vi "Write.vi"(7 "Input String":string, 8 "error in (no error)":errorcluster, 11 "VISA resource name":refnum<visa-resource-name>) -> (0 "error out":errorcluster, 2 "String":string, 3 "VISA resource name out":refnum<visa-resource-name>)   [LabVIEW 2021, in "BK Precision 169XB.lvlib"]
uses:
  BK Precision 169XB.lvlib
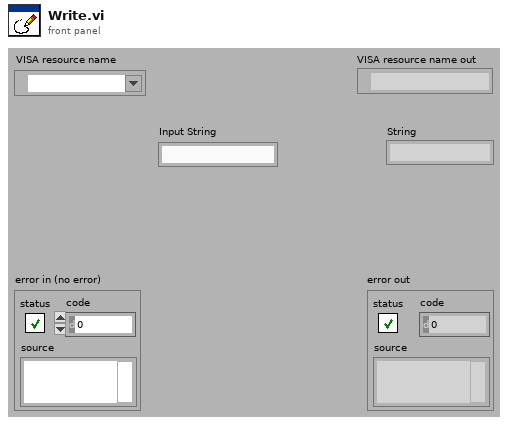
[diagram p1: front panel]
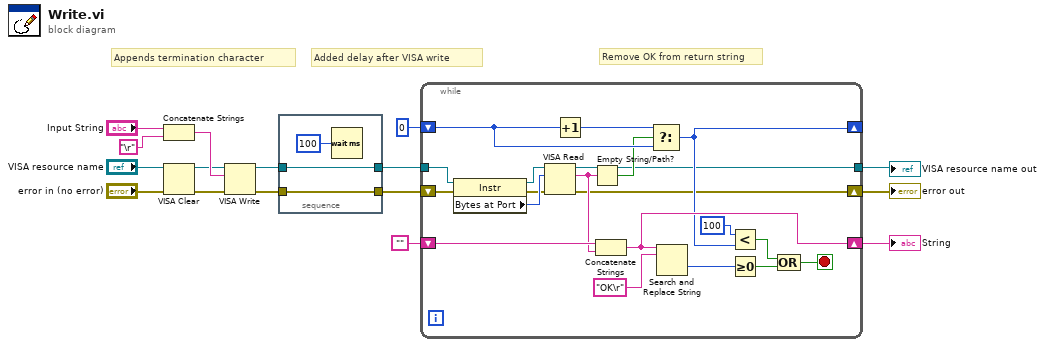
[diagram p0: block diagram]
diagram:
  # "Remove OK from return string"
  # "Appends termination character"
  # "Added delay after VISA write"
  n1 = Concatenate Strings("Input String", "\r" ("Carriage Return Constant")) -> (w12:string)
  n2 = VISA Clear(VISA resource name="VISA resource name", error in (no error)="error in (no error)") -> (VISA resource name out=w9:refnum<visa-resource-name>, error out=w10:errorcluster)
  n3 = VISA Write(VISA resource name=w9, write buffer=w12, error in (no error)=w10) -> (VISA resource name out=w8:refnum<visa-resource-name>, error out=w15:errorcluster)  [unwired: 1 out]
  n4 = stacked-sequence {
    tunnel: [w19] -> w14
    tunnel: w15 -> [w19]
    tunnel: w8 -> [w17]
    tunnel: [w17] -> w7
    frame #0 {
      n5 = Wait (ms)(milliseconds to wait=u32 100) -> ()  [unwired: 1 out]
    }
  }
  n6 = while {
    tunnel: [w21] -> w6
    shift-right: [w33] -> w1
    shift-left: "" -> [w35]
    shift-right: [w24] -> _
    shift-left: 0 -> [w23]
    shift-right: [w20] -> w5
    shift-left: w14 -> [w39]
    tunnel: w7 -> [w28]
    stop <- w34 stop-if-true
    n7 = property class="Instr"(reference=w28, error in=w39) -> (reference out=w38:refnum<visa-resource-name>, error out=w36:errorcluster, "Bytes at Port"=w37:u32)
    n8 = VISA Read(VISA resource name=w38, byte count=w37, error in (no error)=w36) -> (VISA resource name out=w21:refnum<visa-resource-name>, read buffer=w29:string, error out=w20:errorcluster)  [unwired: 1 out]
    n9 = Increment(x=w23) -> (x+1=w25:i32)
    n10 = Empty String/Path?(string/path=w29) -> (empty?=w22:bool)
    n11 = Concatenate Strings(w35, w29) -> (w33:string)
    n12 = Select(t=w25, s=w22, f=w23) -> (s? t:f=w24:i32)
    n13 = Search and Replace String(input string=w33, search string="OK\r" ("y")) -> (offset past replacement=w31:i32)  [unwired: 6 in, 3 out]
    n14 = Less?(x=100, y=w24) -> (x < y?=w27:bool)
    n15 = Greater Or Equal To 0?(x=w31) -> (x >= 0?=w26:bool)
    n16 = Compound Arithmetic op=OR(w27, w26) -> (w34:bool)
  }
  "error out" <- w5
  "VISA resource name out" <- w6
  "String" <- w1
